vi "Main.vi"(11 "Module Admin":refnum<class "Delacor_lib_QMH_Cloneable Module Admin.lvclass">) -> ()   [LabVIEW 2025, in "USB IO.lvlib"]
doc: "This template is based off of the Queued Message Handler design pattern and the Queued Message Handler project template that ships with LabVIEW.\n\nThe main difference is that the queue is private to this module and communication between modules is performed via Broadcast and Request events.\n\nRequest events are wrapped in public API methods and are handled in the Event Handling Loop (EHL) of this VI. Any module can register for Broadcast events sent by this module. The EHL generates messages based on user interface actions.\n\nThe Message Handling Loop (MHL) processes messages generated by the EHL, or by other messages. The messages are string values, so new messages can be added easily to the Message Cases case structure in the MHL. Each message cluster can also provide an optional value for Message Data, which is a variant that can be converted to whatever message-specific data is required.\n_____\nBased on DQMH Dev Tools: Project Template 7.1.2.1547."
uses:
  USB IO.lvlib
  <vilib>/Delacor/Delacor QMH/Libraries/Cloneable Module Admin_class/Delacor_lib_QMH_Cloneable Module Admin.lvclass
  Module Data--cluster.ctl
  torque-test-station/Classes/USB IO/USB IO.lvclass
  <vilib>/Delacor/Delacor QMH/Libraries/Message Queue_class/Delacor_lib_QMH_Message Queue.lvclass/Delacor_lib_QMH_Message Queue.ctl
  <vilib>/Delacor/Delacor QMH/Libraries/Cloneable Module Admin_class/Delacor_lib_QMH_Cloneable Module Admin.lvclass/Delacor_lib_QMH_Cloneable Module Admin.ctl
  Stop Argument--cluster.ctl
  <vilib>/Delacor/Delacor QMH/Libraries/Module Admin_class/Delacor_lib_QMH_Module Admin.lvclass/Delacor_lib_QMH_Module Admin.ctl
  read config Argument--cluster.ctl
  init Argument--cluster.ctl
  init (Reply Payload)--cluster.ctl
  close Argument--cluster.ctl
  write relay Argument--cluster.ctl
  torque-test-station/Classes/USB IO/Relay Line.ctl
  write relay (Reply Payload)--cluster.ctl
  <vilib>/Utility/miscctls.llb/LVPointTypeDef.ctl
  <vilib>/Delacor/Delacor QMH/Libraries/Message Queue_class/Delacor_lib_QMH_Enqueue Message (Single).vi
  <vilib>/Delacor/Delacor QMH/Libraries/Cloneable Module Admin_class/Delacor_lib_QMH_Get Module ID.vi
  <vilib>/Delacor/Delacor QMH/Libraries/Module Admin_class/Delacor_lib_QMH_Get External Launch.vi
  <vilib>/Delacor/Delacor QMH/Libraries/Message Queue_class/Delacor_lib_QMH_Message Queue.lvclass
panel:
  out "error out":errorcluster
  out "Status":string
  in  "Simulate EHL Error":bool
  in  "Simulate MHL Error":bool
  # "Other processes communicate with this Module via its Public API (wrappers for its Request Events).\n\nThis Module communicates with other processes via its Broadcast Events.\nAny process that wants to receive these messages can register for this module's Broadcast events."
  # "This template is for the DQMH framework. See the block diagram for more information on how to use this template."
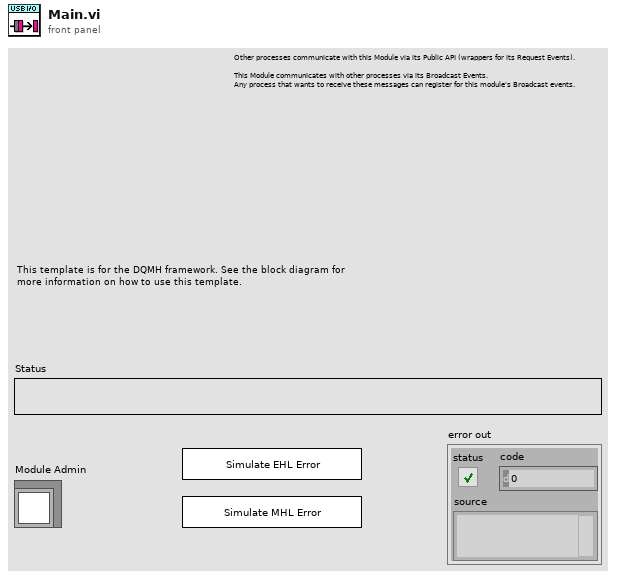
[diagram p1: front panel]
types:
  T1 = typedef "USB IO.lvlib/Request Events--cluster.ctl" = cluster{"Stop Module":refnum<user-event>, "Show Panel":refnum<user-event>, "Hide Panel":refnum<user-event>, "Show Diagram":refnum<user-event>, "Get Module Execution Status":refnum<user-event>, "read config":refnum<user-event>, "init":refnum<user-event>, "close":refnum<user-event>, "write relay":refnum<user-event>}
  T2 = typedef "USB IO.lvlib/Module Data--cluster.ctl" = cluster{"Status":string, "USB IO Object":refnum<class "USB IO.lvclass">}
  T3 = enum32{"invalid lock state", "Not Locked", "Locked (No Password)", "Password-protected"}
  T4 = typedef "USB IO.lvlib/Stop Argument--cluster.ctl" = cluster{"Module ID":i32, "Origin":string, "Exit via Stop Module Req?":bool, "Wait for Module to stop?":bool}
  T5 = typedef "USB IO.lvlib/read config Argument--cluster.ctl" = cluster{"Module ID":i32, "config file path":path}
  T6 = typedef "USB IO.lvlib/init Argument--cluster.ctl" = cluster{"Module ID":i32, "Wait Notifier":refnum<notifier>, "wait for reply":bool}
  T7 = typedef "USB IO.lvlib/close Argument--cluster.ctl" = cluster{"Module ID":i32, "Boolean":bool}
  T8 = typedef "USB IO.lvlib/write relay Argument--cluster.ctl" = cluster{"Module ID":i32, "Line Enum":T9, "High/Low":bool, "Wait Notifier":refnum<notifier>, "wait for reply":bool}
  T9 = typedef "Relay Line.ctl" = enum16{"Brake Relay", "PS Relay"}
  T10 = typedef "LVPointTypeDef.ctl" = cluster{"Horizontal":i16, "Vertical":i16}
  T11 = enum32{"Invalid", "Standard", "Closed", "Hidden", "Minimized", "Maximized"}
  T12 = typedef "USB IO.lvlib/init (Reply Payload)--cluster.ctl" = cluster{"Module ID":i32, "error":errorcluster}
  T13 = typedef "USB IO.lvlib/write relay (Reply Payload)--cluster.ctl" = cluster{"Module ID":i32, "error":errorcluster}
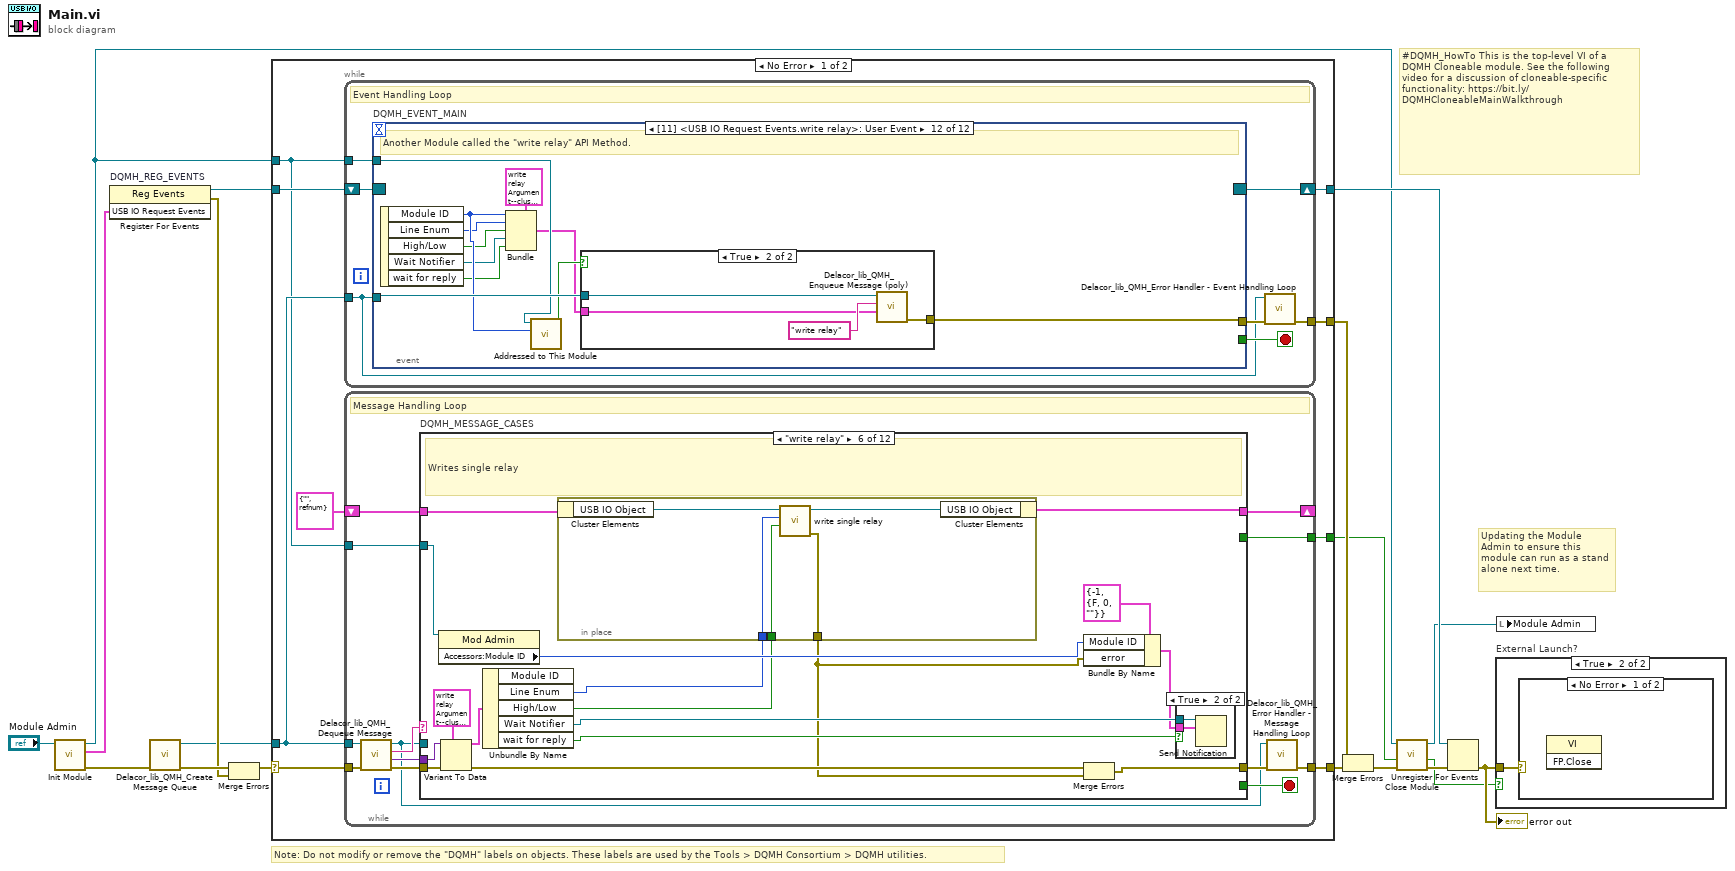
[diagram p0: block diagram]
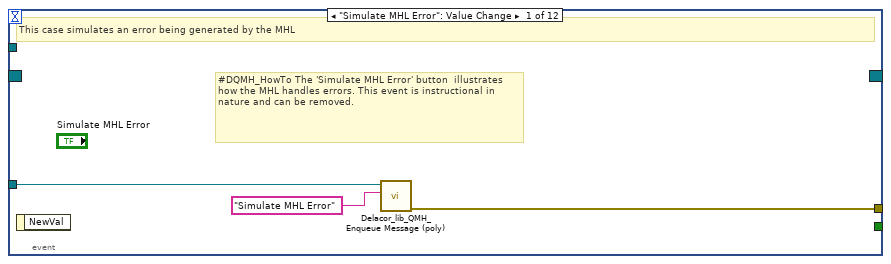
[diagram p2: hidden frame]
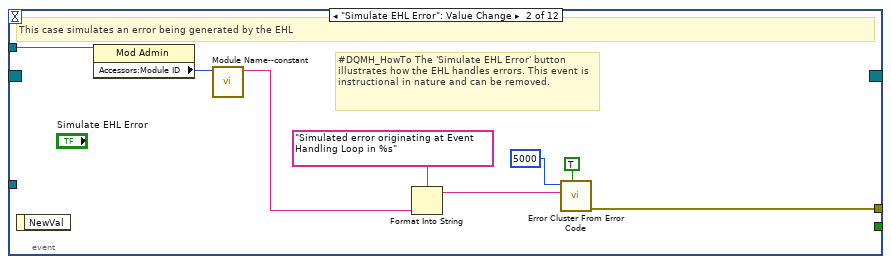
[diagram p3: hidden frame]
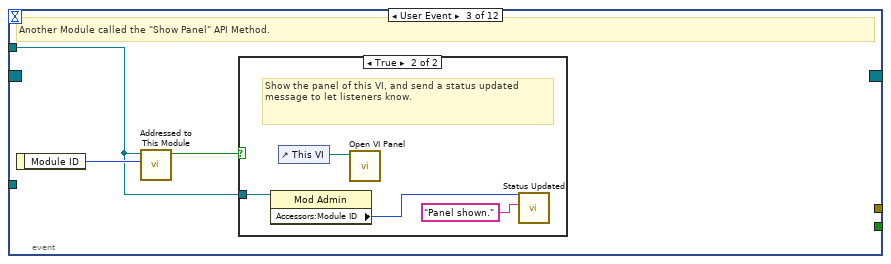
[diagram p4: hidden frame]
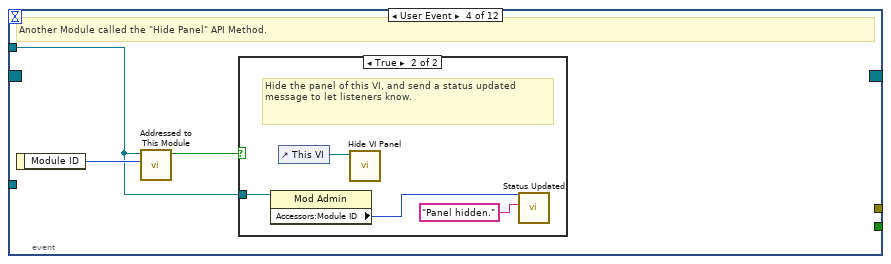
[diagram p6: hidden frame]
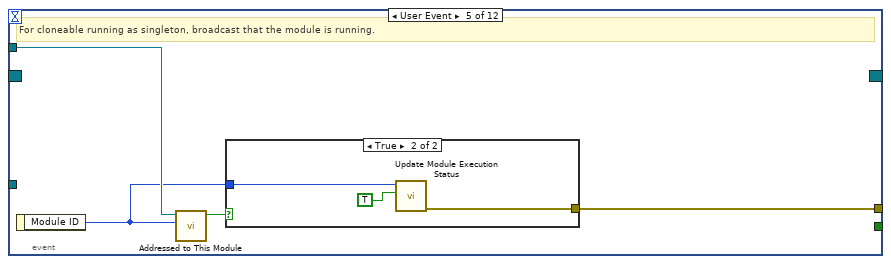
[diagram p8: hidden frame]
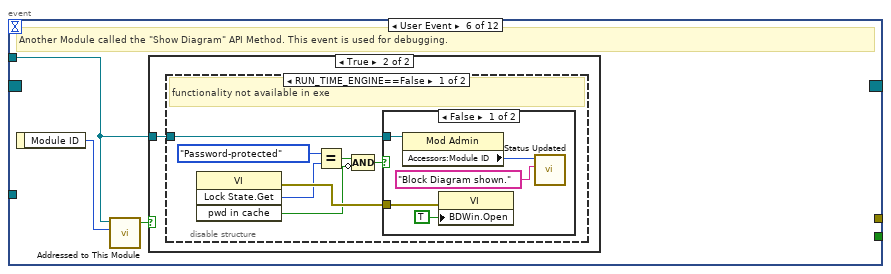
[diagram p10: hidden frame]
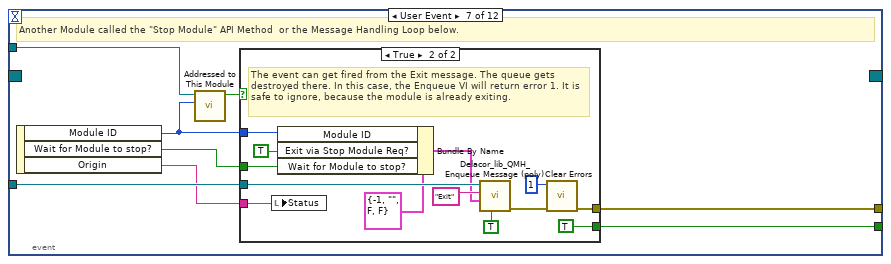
[diagram p14: hidden frame]
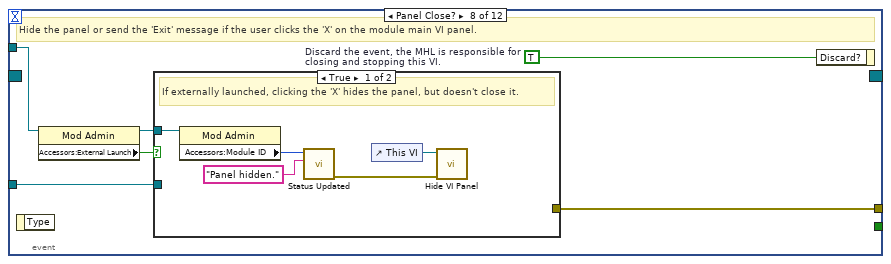
[diagram p16: hidden frame]
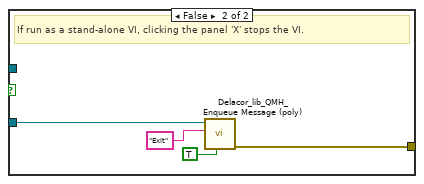
[diagram p17: hidden frame]
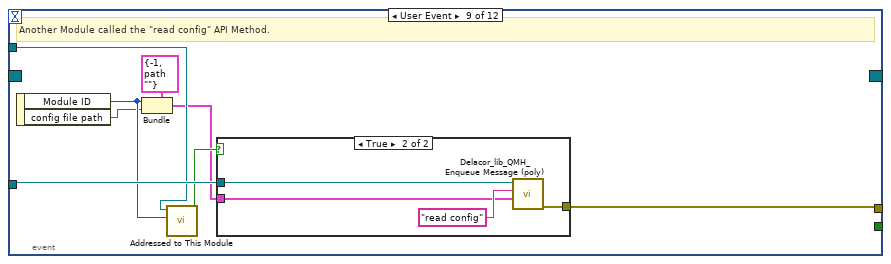
[diagram p18: hidden frame]
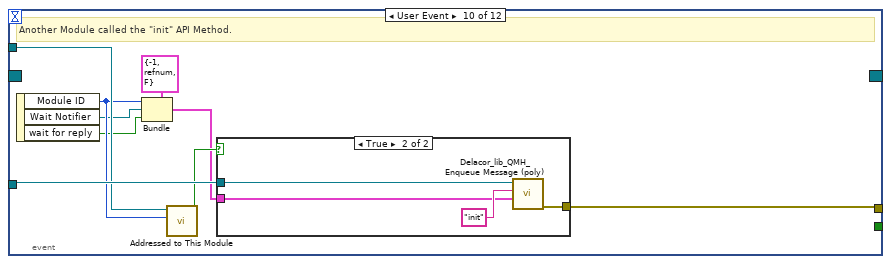
[diagram p20: hidden frame]
diagram:
  # "#DQMH_HowTo This is the top-level VI of a DQMH Cloneable module. See the following video for a discussion of cloneable-specific functionality: https://bit.ly/DQMHCloneableMainWalkthrough"
  # "Note: Do not modify or remove the \"DQMH\" labels on objects. These labels are used by the Tools > DQMH Consortium > DQMH utilities."
  # "Updating the Module Admin to ensure this module can run as a stand alone next time."
  n1 = call "Init Module.vi"("Cloneable Module Admin in"="Module Admin") -> ("error out"=w15:errorcluster, "USB IO Request Events"=w7:T1, "Cloneable Module Admin out"=w4:refnum<class "Delacor_lib_QMH_Cloneable Module Admin.lvclass">)  [unwired: 8 in]
  n2 = register-events "DQMH_REG_EVENTS"(w7) -> (reference out=w8:refnum<event-registration>, error out=w10:errorcluster)  [unwired: 2 in]
  n3 = call <vilib>:"Delacor_lib_QMH_Create Message Queue.vi"("error in"=w15) -> ("error out"=w12:errorcluster, "Message Queue"=w6:refnum<class "Delacor_lib_QMH_Message Queue.lvclass">)  [unwired: 9 in]
  n4 = Merge Errors(w12, w10) -> (w11:errorcluster)
  n5 = case shown="No Error" w11 {
    selector: w11 -> [w25 w349]
    tunnel: [w27 w348] -> w16
    tunnel: [w24 w347] -> w9
    tunnel: w8 -> [w22 w347]
    tunnel: w6 -> [w21 w340]
    tunnel: [w26 _] -> w17
    tunnel: w4 -> [w20 w343]
    tunnel: [w19 _] -> w2
    frame No Error {
      n6 = while {
        tunnel: w21 -> [w28]
        shift-right: [w31] -> w24
        shift-left: w22 -> [w32]
        tunnel: [w33] -> w26
        tunnel: w20 -> [w29]
        stop <- w30 stop-if-true
        # "Event Handling Loop"
        n7 = event "DQMH_EVENT_MAIN" shown="[11] <USB IO Request Events.write relay>: User Event" {
          selector: w32 -> [_ _ _ _ _ _ _ _ _ _ _ _]
          dyn-events: [_ _ _ _ _ _ _ _ _ _ _ _] -> w31
          timeout: _ -> [_ _ _ _ _ _ _ _ _ _ _ _]
          tunnel: [_ _ _ _ _ _ w86 _ _ _ _ _] -> w30
          tunnel: w28 -> [w36 _ _ _ _ _ w89 w106 w126 w139 w151 w166]
          tunnel: [w37 w45 _ _ w63 _ w90 w109 w119 w131 w144 w156] -> w34
          tunnel: w29 -> [_ w44 w46 w53 w61 w67 w88 w107 w124 w137 w149 w164]
          event "Simulate MHL Error": Value Change {
            # "#DQMH_HowTo The 'Simulate MHL Error' button  illustrates how the MHL handles errors. This event is instructional in nature and can be removed."
            # "This case simulates an error being generated by the MHL"
            n8 = event-data() -> ()  [unwired: 1 in, 1 out]
            n9 = call-poly <vilib>:"Delacor_lib_QMH_Enqueue Message (poly).vi"("Message"="Simulate MHL Error", "Message Queue in"=w36) -> ("error out"=w37:errorcluster)  [unwired: 8 in, 1 out]
          }
          event "Simulate EHL Error": Value Change {
            # "#DQMH_HowTo The 'Simulate EHL Error' button  illustrates how the EHL handles errors. This event is instructional in nature and can be removed."
            # "This case simulates an error being generated by the EHL"
            n10 = event-data() -> ()  [unwired: 1 in, 1 out]
            n11 = property on="Property Node" class="Mod Admin"(reference=w44) -> ("Accessors:Module ID"=w43:i32)  [unwired: 1 in, 2 out]
            n12 = call "Module Name--constant.vi"("Module ID"=w43) -> ("Module Name"=w38:string)  [unwired: 10 in]
            n13 = Format Into String(format string="Simulated error originating at Event Handling Loop in %s", w38) -> (resulting string=w41:string)  [unwired: 2 in, 1 out]
            n14 = call <vilib>:"Error Cluster From Error Code.vi"("show call chain? (False)"=TRUE, "error message (\"\")"=w41, "error code (0)"=5000) -> ("error out"=w45:errorcluster)  [unwired: 6 in]
          }
          event User Event {
            # "Another Module called the \"Show Panel\" API Method."
            n15 = event-data() -> ("Module ID"=w47:i32)  [unwired: 1 in]
            n16 = call "Addressed to This Module.vi"("Module ID from Argument"=w47, "Module Admin"=w46) -> ("Addressed to this instance?"=w48:bool)  [unwired: 8 in, 1 out]
            n17 = case shown="True" w48 {
              tunnel: w46 -> [_ w50]
              frame False {
              }
              frame True {
                # "Show the panel of this VI, and send a status updated message to let listeners know."
                n18 = property on="Property Node" class="Mod Admin"(reference=w50) -> ("Accessors:Module ID"=w49:i32)  [unwired: 1 in, 2 out]
                n19 = control-ref of="This VI"() -> (w52:refnum<vi>)
                n20 = call "Open VI Panel.vi"("VI"=w52) -> ()  [unwired: 10 in, 1 out]
                n21 = call "Status Updated.vi"("Status"="Panel shown." ("format string"), "Module ID"=w49) -> ()  [unwired: 9 in, 1 out]
              }
            }
          }
          event User Event {
            # "Another Module called the \"Hide Panel\" API Method."
            n22 = event-data() -> ("Module ID"=w54:i32)  [unwired: 1 in]
            n23 = call "Addressed to This Module.vi"("Module ID from Argument"=w54, "Module Admin"=w53) -> ("Addressed to this instance?"=w55:bool)  [unwired: 8 in, 1 out]
            n24 = case shown="True" w55 {
              tunnel: w53 -> [_ w57]
              frame False {
              }
              frame True {
                # "Hide the panel of this VI, and send a status updated message to let listeners know."
                n25 = property on="Property Node" class="Mod Admin"(reference=w57) -> ("Accessors:Module ID"=w56:i32)  [unwired: 1 in, 2 out]
                n26 = control-ref of="This VI"() -> (w59:refnum<vi>)
                n27 = call "Hide VI Panel.vi"("VI"=w59) -> ()  [unwired: 10 in, 1 out]
                n28 = call "Status Updated.vi"("Status"="Panel hidden." ("format string"), "Module ID"=w56) -> ()  [unwired: 9 in, 1 out]
              }
            }
          }
          event User Event {
            # "For cloneable running as singleton, broadcast that the module is running."
            n29 = event-data() -> ("Module ID"=w60:i32)  [unwired: 1 in]
            n30 = call "Addressed to This Module.vi"("Module ID from Argument"=w60, "Module Admin"=w61) -> ("Addressed to this instance?"=w62:bool)  [unwired: 8 in, 1 out]
            n31 = case shown="True" w62 {
              tunnel: [_ w66] -> w63
              tunnel: w60 -> [_ w65]
              frame False {
              }
              frame True {
                n32 = call "Update Module Execution Status.vi"("Running?"=TRUE, "Module ID"=w65) -> ("error out"=w66:errorcluster)  [unwired: 9 in]
              }
            }
          }
          event User Event {
            # "Another Module called the \"Show Diagram\" API Method. This event is used for debugging."
            n33 = event-data() -> ("Module ID"=w68:i32)  [unwired: 1 in]
            n34 = call "Addressed to This Module.vi"("Module ID from Argument"=w68, "Module Admin"=w67) -> ("Addressed to this instance?"=w69:bool)  [unwired: 8 in, 1 out]
            n35 = case shown="True" w69 {
              tunnel: w67 -> [_ w70]
              frame False {
              }
              frame True {
                n36 = disable-structure shown="RUN_TIME_ENGINE==False" {
                  disable-tunnel: w70 -> [w71 _]
                  frame condition #0 (active) {
                    # "functionality not available in exe"
                    n37 = invoke on="Invoke Node" class="VI" method="Lock State.Get"() -> (error out=w77:errorcluster, "Get Lock State"=w76:T3, "pwd in cache"=w73:bool)  [unwired: 4 in, 1 out]
                    n38 = Equal?(x=T3."Password-protected", y=w76) -> (x = y?=w74:bool)
                    n39 = Compound Arithmetic op=AND(w74, invert w73) -> (w72:bool)
                    n40 = case shown="False" w72 {
                      tunnel: w77 -> [w82 _]
                      tunnel: w71 -> [w79 _]
                      frame False {
                        n41 = property on="Property Node" class="Mod Admin"(reference=w79) -> ("Accessors:Module ID"=w78:i32)  [unwired: 1 in, 2 out]
                        n42 = property on="Property Node" class="VI"(error in=w82, "BDWin.Open"=TRUE ("Block Diagram Window:Open")) -> ()  [unwired: 1 in, 2 out]
                        n43 = call "Status Updated.vi"("Status"="Block Diagram shown." ("format string"), "Module ID"=w78) -> ()  [unwired: 9 in, 1 out]
                      }
                      frame True {
                        # "Password-protected VI, and the password is not in the cache. Do not show the diagram."
                      }
                    }
                  }
                  frame condition #1 {
                  }
                }
              }
            }
          }
          event User Event {
            # "Another Module called the \"Stop Module\" API Method  or the Message Handling Loop below."
            n44 = event-data() -> ("Module ID"=w84:i32, "Wait for Module to stop?"=w85:bool, "Origin"=w83:string)  [unwired: 1 in]
            n45 = call "Addressed to This Module.vi"("Module ID from Argument"=w84, "Module Admin"=w88) -> ("Addressed to this instance?"=w87:bool)  [unwired: 8 in, 1 out]
            n46 = case shown="True" w87 {
              tunnel: [_ w102] -> w90
              tunnel: w89 -> [_ w98]
              tunnel: [_ TRUE] -> w86
              tunnel: w85 -> [_ w93]
              tunnel: w84 -> [_ w95]
              tunnel: w83 -> [_ w91]
              frame False {
              }
              frame True {
                # "The event can get fired from the Exit message. The queue gets destroyed there. In this case, the Enqueue VI will return error 1. It is safe to ignore, because the module is already exiting."
                n47 = local write "Status"(w91) -> ()
                n48 = Bundle By Name(cluster=T4 {"Module ID"=-1, "Origin"="", "Exit via Stop Module Req?"=FALSE, "Wait for Module to stop?"=FALSE} ("Stop Argument"), "Module ID"=w95, "Exit via Stop Module Req?"=TRUE, "Wait for Module to stop?"=w93) -> (w92:T4)
                n49 = call-poly <vilib>:"Delacor_lib_QMH_Enqueue Message (poly).vi"("Priority Message? (F)"=TRUE, "Message Data"=w92, "Message"="Exit", "Message Queue in"=w98) -> ("error out"=w103:errorcluster)  [unwired: 6 in, 1 out]
                n50 = call <vilib>:"Clear Errors.vi"("error in (no error)"=w103, "specific error code to clear (0: all)"=1) -> ("error out"=w102:errorcluster)  [unwired: 4 in, 1 out]
              }
            }
          }
          event Panel Close? {
            w108 = TRUE  # Discard the event, the MHL is responsible for closing and stopping this VI.
            # "Hide the panel or send the 'Exit' message if the user clicks the 'X' on the module main VI panel."
            n51 = event-data() -> ()  [unwired: 1 in, 1 out]
            n52 = property on="Property Node" class="Mod Admin"(reference=w107) -> (reference out=w104:refnum<class "Delacor_lib_QMH_Cloneable Module Admin.lvclass">, "Accessors:External Launch"=w105:bool)  [unwired: 1 in, 1 out]
            n53 = case shown="True" w105 {
              tunnel: w106 -> [_ w117]
              tunnel: [_ w118] -> w109
              tunnel: w104 -> [w112 _]
              frame True {
                # "If externally launched, clicking the 'X' hides the panel, but doesn't close it."
                n54 = property on="Property Node" class="Mod Admin"(reference=w112) -> ("Accessors:Module ID"=w111:i32)  [unwired: 1 in, 2 out]
                n55 = call "Status Updated.vi"("Status"="Panel hidden." ("format string"), "Module ID"=w111) -> ("error out"=w110:errorcluster)  [unwired: 9 in]
                n56 = control-ref of="This VI"() -> (w114:refnum<vi>)
                n57 = call "Hide VI Panel.vi"("error in"=w110, "VI"=w114) -> ()  [unwired: 9 in, 1 out]
              }
              frame False {
                # "If run as a stand-alone VI, clicking the panel 'X' stops the VI."
                n58 = call-poly <vilib>:"Delacor_lib_QMH_Enqueue Message (poly).vi"("Priority Message? (F)"=TRUE, "Message"="Exit", "Message Queue in"=w117) -> ("error out"=w118:errorcluster)  [unwired: 7 in, 1 out]
              }
            }
            n59 = event-data ("Event Filter Node")("Discard?"=w108) -> ()  [unwired: 1 in, 1 out]
          }
          event User Event {
            # "Another Module called the \"read config\" API Method."
            n60 = event-data() -> ("Module ID"=w121:i32, "config file path"=w120:path)  [unwired: 1 in]
            n61 = Bundle(cluster=T5 {"Module ID"=-1, "config file path"=path ""} ("read config Argument"), "Module ID"=w121, "config file path"=w120) -> (w122:T5)
            n62 = call "Addressed to This Module.vi"("Module ID from Argument"=w121, "Module Admin"=w124) -> ("Addressed to this instance?"=w125:bool)  [unwired: 8 in, 1 out]
            n63 = case shown="True" w125 {
              tunnel: w126 -> [_ w130]
              tunnel: w122 -> [_ w128]
              tunnel: [_ w127] -> w119
              frame False {
              }
              frame True {
                n64 = call-poly <vilib>:"Delacor_lib_QMH_Enqueue Message (poly).vi"("Message Data"=w128, "Message"="read config", "Message Queue in"=w130) -> ("error out"=w127:errorcluster)  [unwired: 7 in, 1 out]
              }
            }
          }
          event User Event {
            # "Another Module called the \"init\" API Method."
            n65 = event-data() -> ("Module ID"=w134:i32, "Wait Notifier"=w133:refnum<notifier>, "wait for reply"=w132:bool)  [unwired: 1 in]
            n66 = Bundle(cluster=T6 {"Module ID"=-1, "Wait Notifier"=refnum, "wait for reply"=FALSE} ("init Argument"), "Module ID"=w134, "Wait Notifier"=w133, "wait for reply"=w132) -> (w135:T6)
            n67 = call "Addressed to This Module.vi"("Module ID from Argument"=w134, "Module Admin"=w137) -> ("Addressed to this instance?"=w138:bool)  [unwired: 8 in, 1 out]
            n68 = case shown="True" w138 {
              tunnel: w139 -> [_ w143]
              tunnel: w135 -> [_ w141]
              tunnel: [_ w140] -> w131
              frame False {
              }
              frame True {
                n69 = call-poly <vilib>:"Delacor_lib_QMH_Enqueue Message (poly).vi"("Message Data"=w141, "Message"="init", "Message Queue in"=w143) -> ("error out"=w140:errorcluster)  [unwired: 7 in, 1 out]
              }
            }
          }
          event User Event {
            # "Another Module called the \"close\" API Method."
            n70 = event-data() -> ("Module ID"=w146:i32, "Boolean"=w145:bool)  [unwired: 1 in]
            n71 = Bundle(cluster=T7 {"Module ID"=-1, "Boolean"=FALSE} ("close Argument"), "Module ID"=w146, "Boolean"=w145) -> (w147:T7)
            n72 = call "Addressed to This Module.vi"("Module ID from Argument"=w146, "Module Admin"=w149) -> ("Addressed to this instance?"=w150:bool)  [unwired: 8 in, 1 out]
            n73 = case shown="True" w150 {
              tunnel: w151 -> [_ w155]
              tunnel: w147 -> [_ w153]
              tunnel: [_ w152] -> w144
              frame False {
              }
              frame True {
                n74 = call-poly <vilib>:"Delacor_lib_QMH_Enqueue Message (poly).vi"("Message Data"=w153, "Message"="close", "Message Queue in"=w155) -> ("error out"=w152:errorcluster)  [unwired: 7 in, 1 out]
              }
            }
          }
          event User Event {
            # "Another Module called the \"write relay\" API Method."
            n75 = event-data() -> ("Module ID"=w161:i32, "Line Enum"=w160:T9, "High/Low"=w159:bool, "Wait Notifier"=w158:refnum<notifier>, "wait for reply"=w157:bool)  [unwired: 1 in]
            n76 = Bundle(cluster=T8 {"Module ID"=-1, "Line Enum"=enum."Brake Relay", "High/Low"=FALSE, "Wait Notifier"=refnum, "wait for reply"=FALSE} ("write relay Argument"), "Module ID"=w161, "Line Enum"=w160, "High/Low"=w159, "Wait Notifier"=w158, "wait for reply"=w157) -> (w162:T8)
            n77 = call "Addressed to This Module.vi"("Module ID from Argument"=w161, "Module Admin"=w164) -> ("Addressed to this instance?"=w165:bool)  [unwired: 8 in, 1 out]
            n78 = case shown="True" w165 {
              tunnel: w166 -> [_ w170]
              tunnel: w162 -> [_ w168]
              tunnel: [_ w167] -> w156
              frame False {
              }
              frame True {
                n79 = call-poly <vilib>:"Delacor_lib_QMH_Enqueue Message (poly).vi"("Message Data"=w168, "Message"="write relay", "Message Queue in"=w170) -> ("error out"=w167:errorcluster)  [unwired: 7 in, 1 out]
              }
            }
          }
        }
        n80 = call-dynamic "Delacor_lib_QMH_Error Handler - Event Handling Loop.vi"("error in"=w34, "Message Queue in"=w28) -> ("dup error in"=w33:errorcluster)  [unwired: 8 in, 1 out]
      }
      n81 = while {
        tunnel: w21 -> [w171]
        shift-right: [w178] -> _
        shift-left: T2 {"Status"="", "USB IO Object"=refnum} ("Data Cluster") -> [w179]
        tunnel: w25 -> [w182]
        tunnel: [w180] -> w27
        tunnel: w20 -> [w173]
        tunnel: [w172] -> w19
        stop <- w177 stop-if-true
        # "Message Handling Loop"
        n82 = call-dynamic "Delacor_lib_QMH_Dequeue Message.vi"("error in"=w182, "Message Queue in"=w171) -> ("error out"=w181:errorcluster, "Message Data"=w175:variant, "Message"=w176:string, "Message Queue out"=w174:refnum<class "Delacor_lib_QMH_Message Queue.lvclass">)  [unwired: 6 in]
        n83 = case "DQMH_MESSAGE_CASES" shown="\"write relay\"" w176 {
          selector: w176 -> [_ _ _ _ _ _ _ _ _ _ _ w329]
          tunnel: w174 -> [_ _ _ _ _ _ _ _ w284 _ w321 _]
          tunnel: w181 -> [w202 w206 w216 w235 w249 w269 w279 w281 w293 w310 w327 w338]
          tunnel: [w200 w206 w207 w226 w241 w260 w278 w281 w289 w309 w322 w339] -> w183
          tunnel: w179 -> [w193 w205 w212 w223 w245 w257 w277 w280 w288 w307 w320 w336]
          tunnel: [w192 w205 w210 w222 w244 w253 w277 w280 w288 w307 w320 w336] -> w178
          tunnel: [_ _ _ _ _ _ _ _ _ _ w319 _] -> w177
          tunnel: w175 -> [_ _ w215 w233 w248 w267 _ _ w287 _ w317 _]
          tunnel: w173 -> [w188 _ _ w224 _ w258 _ _ w286 w305 w312 w335]
          tunnel: [_ _ _ _ _ _ _ _ _ _ w315 _] -> w172
          frame "Initialize" {
            w185 = "Initial Message" ("Initial Message")
            # "#DQMH_CodeNeeded - Initialize the appearance of the front panel."
            # "#DQMH_CodeNeeded - Initialize your state data here."
            # "Initialize - Any operation that needs to be done before the module can receive messages. Synchronize Caller Events.vi will inform Start Module.vi that the module has launched and is ready to receive messages. Module Did Init.vi will broadcast that the module initialized."
            n84 = call "Synchronize Caller Events.vi"("error in"=w202, "Module Admin"=w188) -> ("error out"=w201:errorcluster, "Module Admin out"=w187:refnum<class "Delacor_lib_QMH_Cloneable Module Admin.lvclass">)  [unwired: 8 in]
            n85 = property on="Property Node" class="Mod Admin"(reference=w187) -> ("Accessors:Module ID"=w184:i32, "Accessors:External Launch"=w189:bool)  [unwired: 1 in, 2 out]
            n86 = call "Module Name--constant.vi"("Module ID"=w184) -> ("Module Name"=w197:string)  [unwired: 10 in]
            n87 = property on="Property Node" class="VI"("Front Panel.Title"=w197) -> (reference out=w199:refnum<vi>, error out=w204:errorcluster)  [unwired: 2 in]
            n88 = Select(t=T11."Hidden" ("State"), s=w189, f=T11."Standard" ("State")) -> (s? t:f=w194:T11)
            n89 = invoke on="Invoke Node" class="VI" method="FP.Open"(reference=w199, error in=w204, "State"=w194) -> (reference out=w198:refnum<vi>, error out=w203:errorcluster)  [unwired: 2 in, 3 out]
            n90 = Bundle By Name(cluster=w193, "Status"=w185) -> (w192:T2)
            n91 = invoke on="Invoke Node" class="VI" method="FP.Center"(reference=w198, error in=w203) -> ()  [unwired: 1 in, 3 out]
            n92 = property on="Pane" class="Pane"("Origin"=T10 {"Horizontal"=0, "Vertical"=0}) -> ()  [unwired: 2 in, 2 out]
            n93 = call "Module Name--constant.vi"("Module ID"=w184) -> ("Module Name"=w190:string)  [unwired: 10 in]
            n94 = call "Module Did Init.vi"("error in"=w201, "Initialized?"=TRUE, "Origin"=w190, "Module ID"=w184) -> ("error out"=w200:errorcluster)  [unwired: 7 in]
            "Status" <- w185
          }
          frame "---Module Specific---" {
            # "Separator -- The following cases handle messages specific to this Module."
          }
          frame "read config" {
            # "Reads .json config file to initialize object."
            n95 = Variant To Data(error in=w216, type=T5 {"Module ID"=-1, "config file path"=path ""} ("read config Argument"), Variant=w215) -> (data=w213:T5, error out=w208:errorcluster)
            n96 = Unbundle By Name(w213) -> ("config file path"=w211:path)  [unwired: 1 out]
            n97 = in-place {
              in-place-border: w211 -> [w219]
              in-place-border: [w217] -> w209
              n98 = in-place-cluster #1(w212) -> ("USB IO Object"=w220:refnum<class "USB IO.lvclass">)
              n99 = call-dynamic "read config.vi"("config file path"=w219, "USB IO in"=w220) -> ("error out"=w217:errorcluster, "USB IO out"=w218:refnum<class "USB IO.lvclass">)  [unwired: 8 in]
              n100 = in-place-cluster #1("USB IO Object"=w218) -> (w210:T2)
            }
            n101 = Merge Errors(w209, w208) -> (w207:errorcluster)
          }
          frame "init" {
            # "Initializes DAQmx Channel"
            n102 = property class="Mod Admin"(reference=w224) -> ("Accessors:Module ID"=w225:i32)  [unwired: 1 in, 2 out]
            n103 = Variant To Data(error in=w235, type=T6 {"Module ID"=-1, "Wait Notifier"=refnum, "wait for reply"=FALSE} ("init Argument"), Variant=w233) -> (data=w231:T6, error out=w234:errorcluster)
            n104 = Unbundle By Name(w231) -> ("Wait Notifier"=w230:refnum<notifier>, "wait for reply"=w229:bool)  [unwired: 1 out]
            n105 = in-place {
              in-place-border: [w236] -> w221
              n106 = in-place-cluster #2(w223) -> ("USB IO Object"=w238:refnum<class "USB IO.lvclass">)
              n107 = call-dynamic "init.vi"("USB IO in"=w238) -> ("error out"=w236:errorcluster, "USB IO out"=w237:refnum<class "USB IO.lvclass">)  [unwired: 9 in]
              n108 = in-place-cluster #2("USB IO Object"=w237) -> (w222:T2)
            }
            n109 = Bundle By Name(cluster=T12 {"Module ID"=-1, "error"={"status"=FALSE, "code"=0, "source"=""}} ("init (Reply Payload)"), "Module ID"=w225, "error"=w221) -> (w228:T12)
            n110 = Merge Errors(w234, w221) -> (w226:errorcluster)
            n111 = case "DQMH_FIRE_NOTIFIER" shown="True" w229 {
              tunnel: w230 -> [_ w240]
              tunnel: w228 -> [_ w239]
              frame False {
              }
              frame True {
                n112 = Send Notification(notification=w239, notifier=w240) -> ()  [unwired: 1 in, 2 out]
              }
            }
          }
          frame "close" {
            # "Closes DAQmx Channel"
            n113 = Variant To Data(error in=w249, type=T7 {"Module ID"=-1, "Boolean"=FALSE} ("close Argument"), Variant=w248) -> (data=w246:T7, error out=w242:errorcluster)
            n114 = Unbundle By Name(w246) -> ()  [unwired: 2 out]
            n115 = in-place {
              in-place-border: [w250] -> w243
              n116 = in-place-cluster #3(w245) -> ("USB IO Object"=w252:refnum<class "USB IO.lvclass">)
              n117 = call-dynamic "close.vi"("USB IO in"=w252) -> ("error out"=w250:errorcluster, "USB IO out"=w251:refnum<class "USB IO.lvclass">)  [unwired: 9 in]
              n118 = in-place-cluster #3("USB IO Object"=w251) -> (w244:T2)
            }
            n119 = Merge Errors(w243, w242) -> (w241:errorcluster)
          }
          frame "write relay" {
            # "Writes single relay"
            n120 = property class="Mod Admin"(reference=w258) -> ("Accessors:Module ID"=w259:i32)  [unwired: 1 in, 2 out]
            n121 = Variant To Data(error in=w269, type=T8 {"Module ID"=-1, "Line Enum"=enum."Brake Relay", "High/Low"=FALSE, "Wait Notifier"=refnum, "wait for reply"=FALSE} ("write relay Argument"), Variant=w267) -> (data=w265:T8, error out=w268:errorcluster)
            n122 = Unbundle By Name(w265) -> ("Line Enum"=w256:T9, "High/Low"=w255:bool, "Wait Notifier"=w264:refnum<notifier>, "wait for reply"=w263:bool)  [unwired: 1 out]
            n123 = in-place {
              in-place-border: w256 -> [w273]
              in-place-border: w255 -> [w272]
              in-place-border: [w270] -> w254
              n124 = in-place-cluster #4(w257) -> ("USB IO Object"=w274:refnum<class "USB IO.lvclass">)
              n125 = call-dynamic "write single relay.vi"("High/Low"=w272, "Line Enum"=w273, "USB IO in"=w274) -> ("error out"=w270:errorcluster, "USB IO out"=w271:refnum<class "USB IO.lvclass">)  [unwired: 7 in]
              n126 = in-place-cluster #4("USB IO Object"=w271) -> (w253:T2)
            }
            n127 = Bundle By Name(cluster=T13 {"Module ID"=-1, "error"={"status"=FALSE, "code"=0, "source"=""}} ("write relay (Reply Payload)"), "Module ID"=w259, "error"=w254) -> (w262:T13)
            n128 = Merge Errors(w268, w254) -> (w260:errorcluster)
            n129 = case "DQMH_FIRE_NOTIFIER" shown="True" w263 {
              tunnel: w264 -> [_ w276]
              tunnel: w262 -> [_ w275]
              frame False {
              }
              frame True {
                n130 = Send Notification(notification=w275, notifier=w276) -> ()  [unwired: 1 in, 2 out]
              }
            }
          }
          frame "---Copy This Frame---" {
            # "Duplicate this frame when creating new messages.  Change this comment in the duplicated frame to describe this message."
            n131 = Merge Errors(w279) -> (w278:errorcluster)
          }
          frame "---Exit and Error Handling---" {
            # "Separator - the following cases handle errors and exit messages."
          }
          frame "Error" {
            # "#DQMH_CodeRecommended - If the module is running in standalone mode (External Launch = FALSE), this code will pop up an error dialog and call the 'Exit' message if an error occurs. Add more fine-grained error management here."
            # "Error - Check the error message data and respond accordingly. This message is sent by the \"Error Handler\" VIs at the end of each loop in this application."
            n132 = property on="Property Node" class="Mod Admin"(reference=w286) -> ("Accessors:External Launch"=w285:bool, "Accessors:Module ID"=w283:i32)  [unwired: 1 in, 2 out]
            n133 = Variant To Data(error in=w293, type=errorcluster {"status"=FALSE, "code"=0, "source"=""} ("error constant"), Variant=w287) -> (data=w282:errorcluster, error out=w291:errorcluster)
            n134 = local write "error out"(w282) -> ()
            n135 = call "Error Reported.vi"("Error"=w282, "Module ID"=w283) -> ()  [unwired: 9 in, 1 out]
            n136 = case shown="False" w285 {
              tunnel: [w298 _] -> w290
              tunnel: w284 -> [w296 _]
              tunnel: w282 -> [w297 _]
              frame False {
                n137 = disable-structure shown="Default" {
                  disable-tunnel: w297 -> [w299 _]
                  frame condition #0 (active) {
                    # "If the module is running standalone, then pop up an error dialog and call the \"Exit\" message."
                    n138 = call <vilib>:"Simple Error Handler.vi"("error in (no error)"=w299) -> ()  [unwired: 4 in, 5 out]
                  }
                  frame condition #1 {
                    # "To prevent the Simple Error Handler VI from being loaded (e.g. when deploying to a Real-Time target), add the Conditional Disable Symbol \"DQMH_Disable_SEH\" to your project and set it to TRUE."
                  }
                }
                n139 = call-poly <vilib>:"Delacor_lib_QMH_Enqueue Message (poly).vi"("Priority Message? (F)"=TRUE, "Message"="Exit", "Message Queue in"=w296) -> ("error out"=w298:errorcluster)  [unwired: 7 in, 1 out]
              }
              frame True {
                # "If the module was launched externally, calling the Error Reported broadcast VI is the only action performed by the \"Error\" message. The module's caller can then process the error appropriately."
              }
            }
            n140 = Merge Errors(w291, w290) -> (w289:errorcluster)
          }
          frame "Simulate MHL Error" {
            # "#DQMH_HowTo The 'Simulate MHL Error' button  illustrates how the MHL handles errors. This event is instructional in nature and can be removed."
            # "Simulate an error occurring at the MHL"
            n141 = property on="Property Node" class="Mod Admin"(reference=w305) -> ("Accessors:Module ID"=w306:i32)  [unwired: 1 in, 2 out]
            n142 = call "Module Name--constant.vi"("Module ID"=w306) -> ("Module Name"=w301:string)  [unwired: 10 in]
            n143 = Format Into String(format string="Simulated error originating at Message Handling Loop in %s", w301) -> (resulting string=w302:string)  [unwired: 2 in, 1 out]
            n144 = call <vilib>:"Error Cluster From Error Code.vi"("show call chain? (False)"=TRUE, "error message (\"\")"=w302, "error code (0)"=5001) -> ("error out"=w308:errorcluster)  [unwired: 6 in]
            n145 = Merge Errors(w310, w308) -> (w309:errorcluster)
          }
          frame "Exit" {
            w318 = 91  # 91: not all Exit messages will have an argument
            w319 = TRUE  # Stop the VI
            # "Release the message queue reference"
            # "#DQMH_CodeNeeded - Add any required cleanup code here."
            # "Exit - Exit the application."
            n146 = Variant To Data(error in=w327, type=T4 {"Module ID"=-1, "Origin"="", "Exit via Stop Module Req?"=FALSE, "Wait for Module to stop?"=FALSE} ("Stop Argument"), Variant=w317) -> (data=w314:T4, error out=w323:errorcluster)
            n147 = call <vilib>:"Clear Errors.vi"("error in (no error)"=w323, "specific error code to clear (0: all)"=w318) -> ("error out"=w326:errorcluster)  [unwired: 4 in, 1 out]
            n148 = property on="Property Node" class="Mod Admin"(reference=w312) -> ("Accessors:Module ID"=w311:i32)  [unwired: 1 in, 2 out]
            n149 = control-ref of="This VI"() -> (w313:refnum<vi>)
            n150 = call-dynamic "Delacor_lib_QMH_Release Message Queue.vi"("error in"=w326, "Message Queue"=w321) -> ("error out"=w325:errorcluster)  [unwired: 9 in]
            n151 = call "Handle Exit.vi"("Stop Argument"=w314, "Module Admin in"=w312, "VI reference"=w313) -> ("error out"=w324:errorcluster, "Wait for Stop?"=w315:bool)  [unwired: 7 in]
            n152 = Merge Errors(w325, w324) -> (w322:errorcluster)
            n153 = call "Error Reported.vi"("Error"=w322, "Module ID"=w311) -> ()  [unwired: 9 in, 1 out]
          }
          frame Default {
            # "'Default' case only runs if there is a message that isn't defined in any of the other cases.  Output a programming error."
            n154 = property on="Property Node" class="Mod Admin"(reference=w335) -> ("Accessors:Module ID"=w334:i32)  [unwired: 1 in, 2 out]
            n155 = call "Module Name--constant.vi"("Module ID"=w334) -> ("Module Name"=w328:string)  [unwired: 10 in]
            n156 = Format Into String(format string="The invalid message string \"%s\" was received in the Message Handling Loop for module \"%s\".", w329, w328) -> (resulting string=w331:string)  [unwired: 2 in, 1 out]
            n157 = call <vilib>:"Error Cluster From Error Code.vi"("show call chain? (False)"=TRUE, "error message (\"\")"=w331, "error code (0)"=1) -> ("error out"=w337:errorcluster)  [unwired: 6 in]
            n158 = Merge Errors(w338, w337) -> (w339:errorcluster)
          }
        }
        n159 = call-dynamic "Delacor_lib_QMH_Error Handler - Message Handling Loop.vi"("error in"=w183, "Message Queue in"=w174) -> ("dup error in"=w180:errorcluster)  [unwired: 8 in, 1 out]
      }
    }
    frame Error {
      n160 = call "Synchronize Caller Events.vi"("Module Admin"=w343) -> ("Module Admin out"=w342:refnum<class "Delacor_lib_QMH_Cloneable Module Admin.lvclass">)  [unwired: 9 in, 1 out]
      n161 = property on="Property Node" class="Mod Admin"(reference=w342) -> ("Accessors:Module ID"=w341:i32)  [unwired: 1 in, 2 out]
      n162 = call-dynamic "Delacor_lib_QMH_Release Message Queue.vi"("error in"=w349, "Message Queue"=w340) -> ("error out"=w348:errorcluster)  [unwired: 9 in]
      n163 = call "Module Name--constant.vi"("Module ID"=w341) -> ("Module Name"=w346:string)  [unwired: 10 in]
      n164 = Format Into String(format string="An error occurred during initialization. %s is no longer running.", w346) -> (resulting string=w344:string)  [unwired: 2 in, 1 out]
      n165 = call "Error Reported.vi"("Additional Information"=w344, "Error"=w348, "Module ID"=w341) -> ()  [unwired: 8 in, 1 out]
    }
  }
  n166 = Merge Errors(w17, w16) -> (w18:errorcluster)
  n167 = call "Close Module.vi"("error in"=w18, "Wait for stop?"=w2, "Module Admin in"=w4) -> ("error out"=w14:errorcluster, "External Launch"=w1:bool, "Module Admin out"=w3:refnum<class "Delacor_lib_QMH_Cloneable Module Admin.lvclass">)  [unwired: 6 in]
  n168 = Unregister For Events(event registration refnum=w9, error in=w14) -> (error out=w13:errorcluster)
  "error out" <- w13
  n169 = case "External Launch?" shown="True" w1 {
    tunnel: w13 -> [_ w350]
    frame False {
    }
    frame True {
      n170 = case shown="No Error" w350 {
        frame No Error {
          n171 = invoke class="VI" method="FP.Close"() -> ()  [unwired: 3 in, 3 out]
        }
        frame Error {
          n172 = disable-structure shown="Default" {
            frame condition #0 (active) {
              n173 = invoke class="VI" method="FP.Open"("Activate"=TRUE ("Activate?")) -> ()  [unwired: 4 in, 5 out]
            }
            frame condition #1 {
              # "Don't show panel on error if running inside a built EXE."
            }
          }
        }
      }
    }
  }
  n174 = local write "Module Admin"(w3) -> ()
